vi "uService GUI.vi"(8 "error in (no error)":errorcluster, 11 "uService Template in":refnum<class "Simple Device Manager.lvclass">) -> (3 "uService Template out":refnum<class "Simple Device Manager.lvclass">)   [LabVIEW 2020, in "Simple Device Manager.lvlib" / "Simple Device Manager.lvclass"]
uses:
  Simple Device Manager.lvclass
  C:/LabVIEW Code/aegis-labview-code/TALOS/TALOS_PPL.lvlibp/Father of all uServices/Father of all uServices/Father of all uServices.lvclass
  TALOS/TALOS_PPL.lvlibp/Father of all uServices/Father of all uServices/Father of all uServices.lvclass
panel:
  out "Device status":bool
  out "Connection":bool
  in  "Check connection":bool
  in  "Current to set":dbl caption="Current"
  out "Temperature":dbl
  out "Current":dbl
  out "Temperature graph":dbl(graph)
  in  "stop New uService":bool
  in  "Set":bool
  # "Virtual Device Manager"
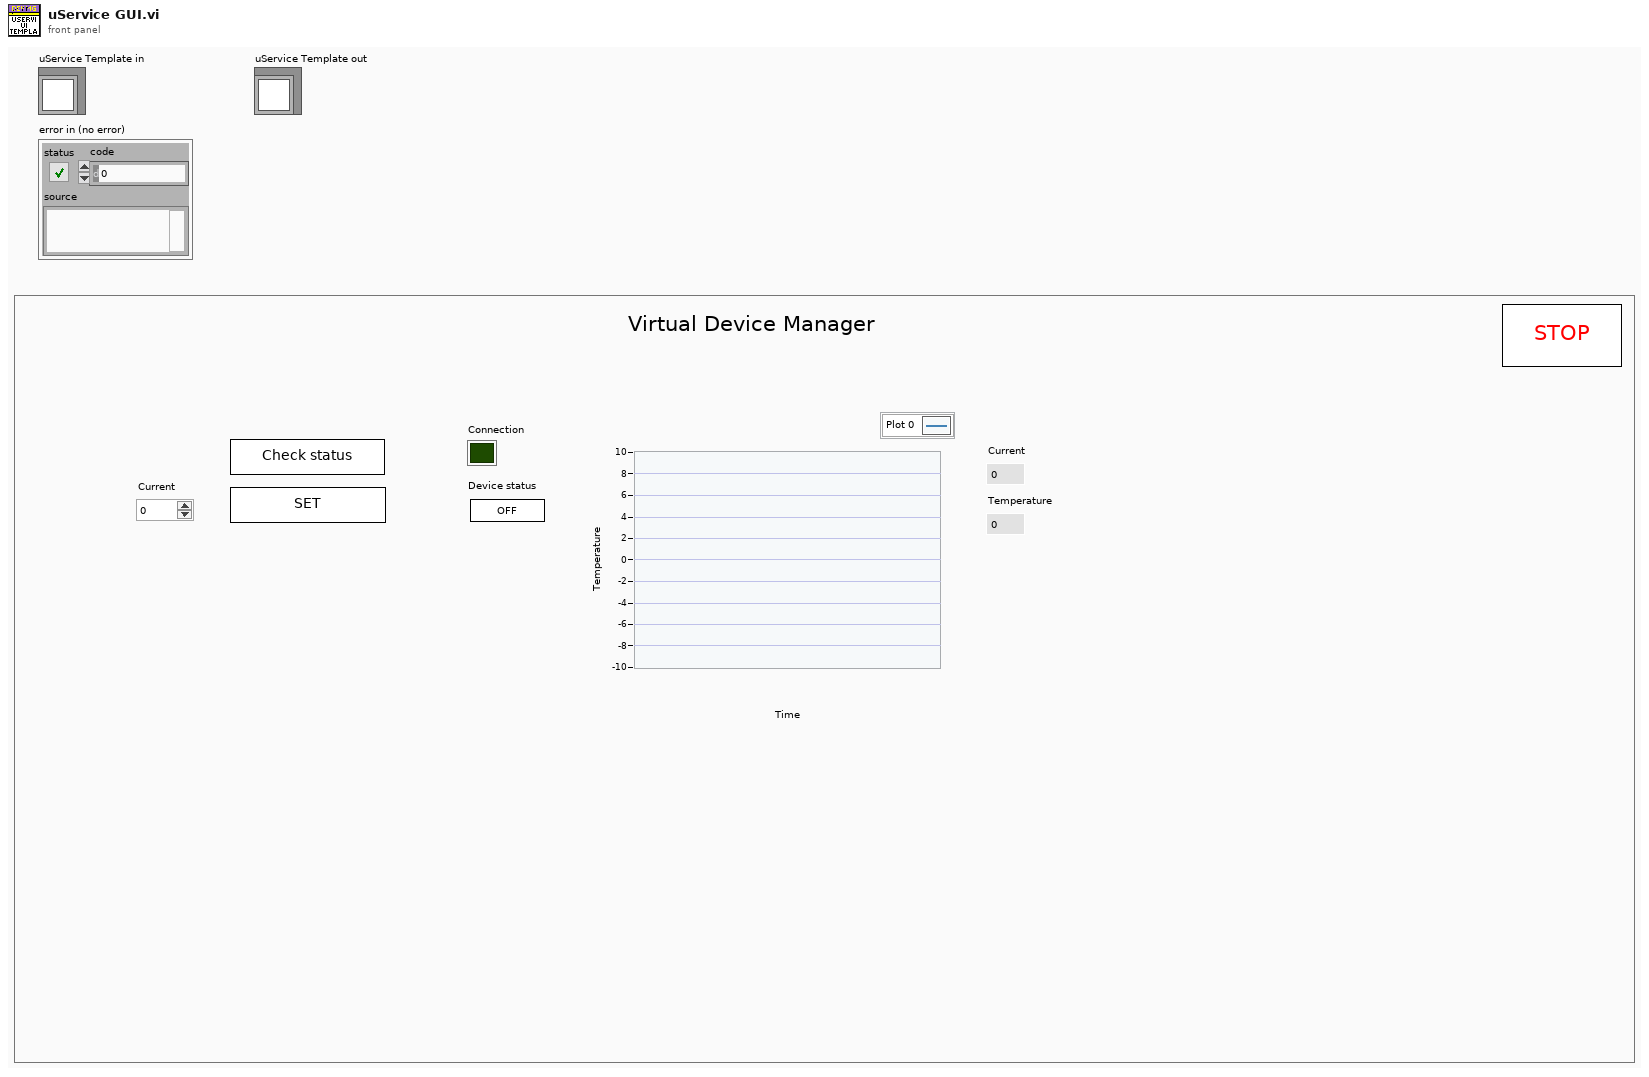
[diagram p1: front panel]
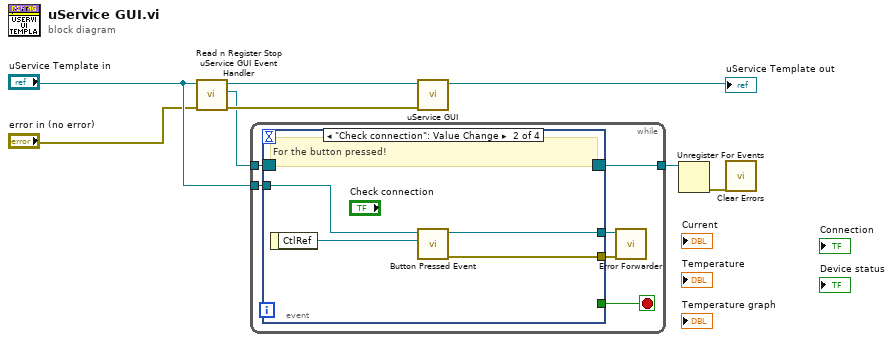
[diagram p0: block diagram]
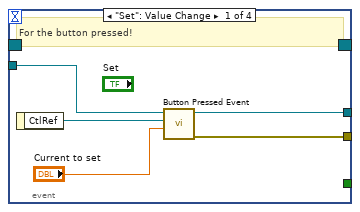
[diagram p2: hidden frame]
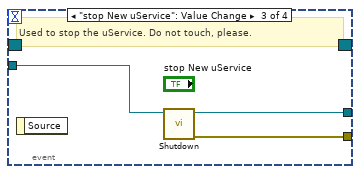
[diagram p3: hidden frame]
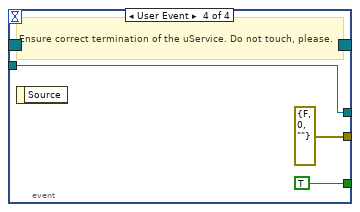
[diagram p4: hidden frame]
diagram:
  n1 = call-dynamic "Read n Register Stop uService GUI Event Handler .vi"("error in (no error)"="error in (no error)", "uService Template in"="uService Template in") -> ("error out"=w6:errorcluster, "Stop uService GUI Event Ref"=w5:refnum<event-registration>, "uService Template out"=w7:refnum<class "Simple Device Manager.lvclass">)  [unwired: 7 in]
  n2 = while {
    tunnel: [w14] -> w8
    tunnel: w5 -> [w12]
    tunnel: "uService Template in" -> [w11]
    stop <- w13 stop-if-true
    n3 = event shown="[1] \"Check connection\": Value Change" {
      selector: w12 -> [_ _ _ _]
      dyn-events: [_ _ _ _] -> w14
      timeout: _ -> [_ _ _ _]
      tunnel: [_ _ _ TRUE] -> w13
      tunnel: w11 -> [w19 w23 w26 w28]
      tunnel: [w17 w21 w25 errorcluster {"status"=FALSE, "code"=0, "source"=""} ("error out")] -> w10
      tunnel: [w16 w20 w24 w28] -> w9
      event "Set": Value Change {
        # "For the button pressed!"
        n4 = event-data() -> ("CtlRef"=w18:refnum<vi>)  [unwired: 1 in]
        n5 = call-dynamic "Button Pressed Event.vi"("Data"="Current to set", "CtlRef"=w18, "uService Template in"=w19) -> ("error out"=w17:errorcluster, "uService Template out"=w16:refnum<class "Simple Device Manager.lvclass">)  [unwired: 7 in]
      }
      event "Check connection": Value Change {
        # "For the button pressed!"
        n6 = event-data() -> ("CtlRef"=w22:refnum<vi>)  [unwired: 1 in]
        n7 = call-dynamic "Button Pressed Event.vi"("CtlRef"=w22, "uService Template in"=w23) -> ("error out"=w21:errorcluster, "uService Template out"=w20:refnum<class "Simple Device Manager.lvclass">)  [unwired: 8 in]
      }
      event "stop New uService": Value Change {
        # "Used to stop the uService. Do not touch, please."
        n8 = event-data() -> ()  [unwired: 1 in, 1 out]
        n9 = call "Shutdown.vi"("Father of all uServices in"=w26) -> ("error out"=w25:errorcluster, "Father of all uServices out"=w24:refnum<class "Simple Device Manager.lvclass">)  [unwired: 9 in]
      }
      event User Event {
        # "Ensure correct termination of the uService. Do not touch, please."
        n10 = event-data() -> ()  [unwired: 1 in, 1 out]
      }
    }
    n11 = call "Error Forwarder.vi"("error in (no error)"=w10, "Father of all uServices in"=w9) -> ()  [unwired: 10 in]
  }
  n12 = call-parent "uService GUI.vi"("error in (no error)"=w6, "uService Template in"=w7) -> ("uService Template out"=→"uService Template out":refnum<class "Simple Device Manager.lvclass">)  [unwired: 9 in]
  n13 = Unregister For Events(event registration refnum=w8) -> (error out=w1:errorcluster)  [unwired: 1 in]
  n14 = call <vilib>:"Clear Errors.vi"("error in (no error)"=w1) -> ()  [unwired: 5 in, 2 out]
